vi "TwoBallAuto2safeTerminal.vi"() -> ()   [LabVIEW 2020]
uses:
  Global Variables/AutoOneBall.ctl
  Global Variables/ActuatorsSensors.vi
  <vilib>/Rock Robotics/WPI/ThirdParty/REV Robotics/REVLib/Typedef/Spark MAX Control Type.ctl
  Global Variables/Axes_N_Buttons.vi
panel:
  in  "Tab Control":T1(tab)=enum."Return Tarmac"
  out "R Output":cluster{"Applied Output":dbl}(graph)
  out "L Output":cluster{"Applied Output":dbl}(graph)
  out "PID R":cluster{"Sensor Position":dbl, "Setpoint":dbl}(graph)
  out "PID L":cluster{"Sensor Position":dbl, "Setpoint":dbl}(graph)
  in  "Reset":bool
  in  "PID Constants L":T2={"P Gain"=0.007, "I Gain"=0.0002, "D Gain"=0.0, "F Gain"=0.0, "I Zone"=1000.0, "Min Output"=-1.0, "Max Output"=1.0}
  in  "PID Constants R":T2={"P Gain"=0.003, "I Gain"=0.0002, "D Gain"=0.0, "F Gain"=0.0, "I Zone"=1000.0, "Min Output"=-0.1, "Max Output"=0.1}
  in  "Range":cluster{"output high":dbl, "output low":dbl}={"output high"=0.6, "output low"=-0.6} {"output low" format="%.2f"; "output high" format="%.2f"}
  in  "Gains":T3={"proportional gain (Kc)"=0.04, "integral time (Ti, min)"=0.0, "derivative time (Td, min)"=0.0} {"derivative time (Td, min)" format="%.3f"; "integral time (Ti, min)" format="%.3f"; "proportional gain (Kc)" format="%.3f"}
  in  "Soft start":dbl=1.8 format="%#_13g"
  in  "Meters":dbl=-2.5
  in  "Meters 2":dbl=2.3
  in  "Meters 3":dbl=-0.6
  in  "Meters 4":dbl=-0.6
  in  "Meters 5":dbl=-1.5
  in  "Meters 6":dbl=-1.0
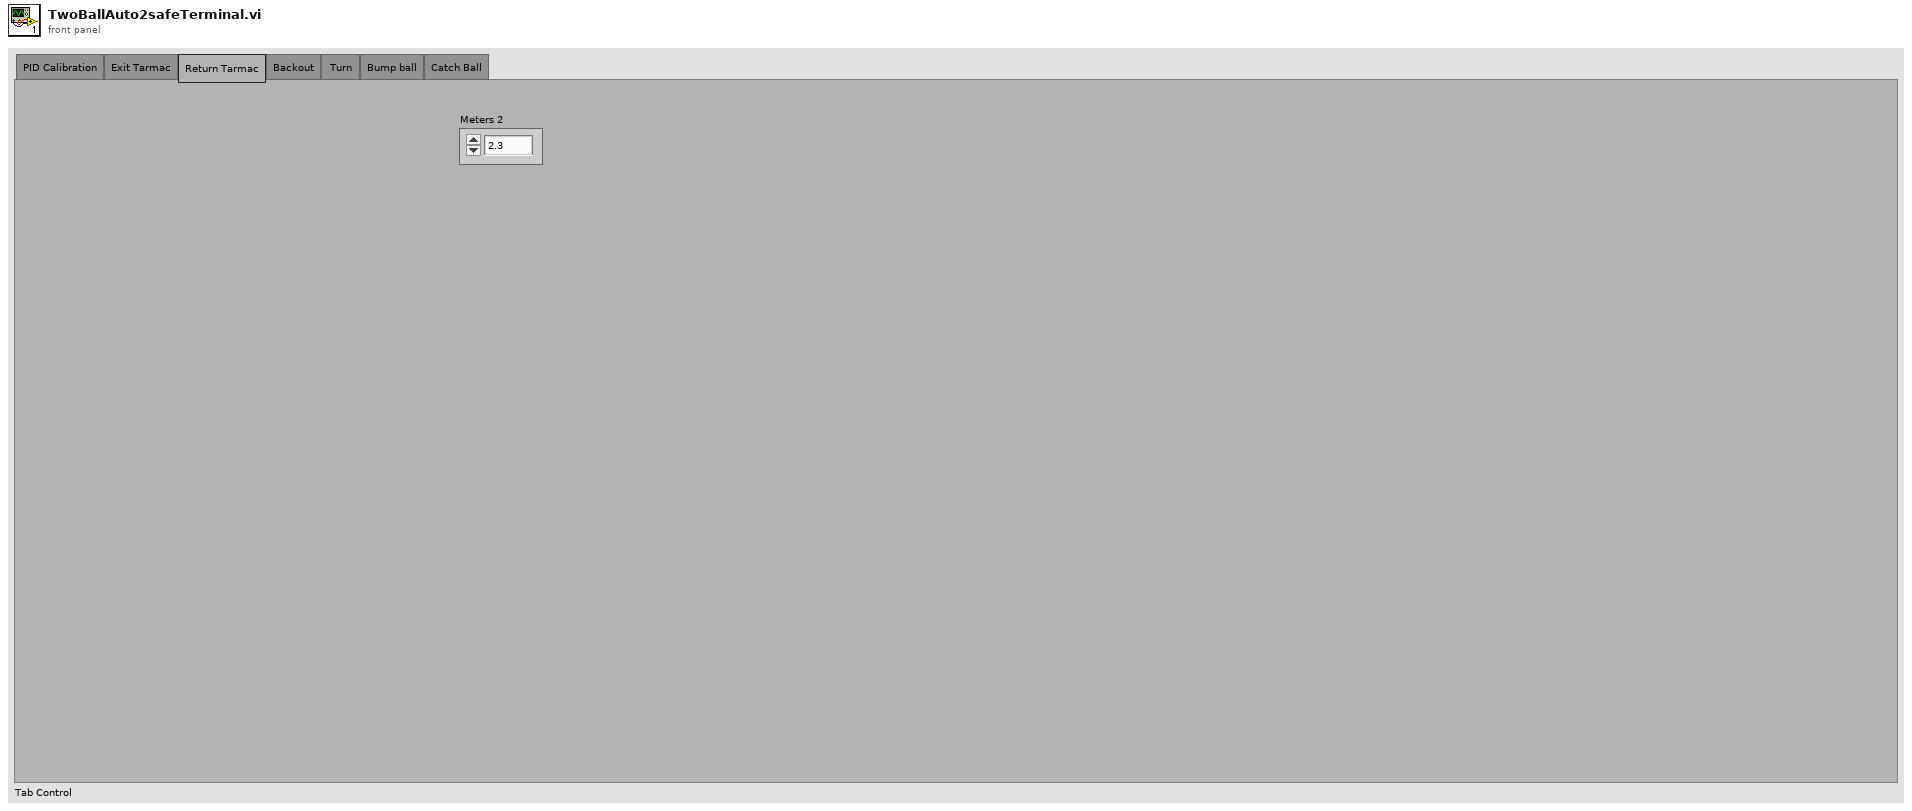
[diagram p1: front panel]
types:
  T1 = enum32{"PID Calibration", "Exit Tarmac", "Return Tarmac", "Backout", "Turn ", "Bump ball", "Catch Ball"}
  T2 = cluster{"P Gain":dbl, "I Gain":dbl, "D Gain":dbl, "F Gain":dbl, "I Zone":dbl, "Min Output":dbl, "Max Output":dbl}
  T3 = cluster{"proportional gain (Kc)":dbl, "integral time (Ti, min)":dbl, "derivative time (Td, min)":dbl}
  T4 = typedef "AutoOneBall.ctl" = enum16{"Start", "Shoot", "Delay", "Exit Tarmac", "Delay 2", "Return Tarmac", "Delay 3", "Prepare Shooter 2", "Align", "Shoot 2", "Backout", "Delay 4", "Turn", "Delay 5", "Bump Ball", "Collect Ball", "Reset"}
  T5 = typedef "WPI_MotorControlDeviceRef.ctl" = cluster{"DeviceStatus":errorcluster, "Type":T6, "PWM":cluster{"PWM Channel":T7, "DeadBand":T8}, "CAN":cluster{"Device Number":u8, "SetOutput VI Ref":variant, "GetOutput VI Ref":variant, "Enable VI Ref":variant, "Disable VI Ref":variant, "Data":variant}, "Invert":bool, "DIO PWM":cluster{"PWM \"Enable\" Channel":T7, "DIOChannel":T9, "PWM Rate":dbl}}
  T6 = typedef "WPI_MotorControlType.ctl" = enum16{"PWM", "CAN", "DIO PWM"}
  T7 = typedef "FPGA_DIOPWMChannel.ctl" = enum8{"PWM 0", "PWM 1", "PWM 2", "PWM 3", "PWM 4", "PWM 5", "PWM 6", "PWM 7", "PWM 8", "PWM 9", "PWM MXP 0", "PWM MXP 1", "PWM MXP 2", "PWM MXP 3", "PWM MXP 4", "PWM MXP 5", "PWM MXP 6", "PWM MXP 7", "PWM MXP 8", "PWM MXP 9", "Invalid"}
  T8 = typedef "WPI_PWMDeadband.ctl" = cluster{"Name":string, "maxPositivePwm":i32, "minPositivePwm":i32, "centerPwm":i32, "maxNegativePwm":i32, "minNegativePwm":i32, "angularRange":u16}
  T9 = typedef "FPGA_DIOChannel.ctl" = enum8{"DIO 0", "DIO 1", "DIO 2", "DIO 3", "DIO 4", "DIO 5", "DIO 6", "DIO 7", "DIO 8", "DIO 9", "DIO MXP 0", "DIO MXP 1", "DIO MXP 2", "DIO MXP 3", "DIO MXP 4", "DIO MXP 5", "DIO MXP 6", "DIO MXP 7", "DIO MXP 8", "DIO MXP 9", "DIO MXP 10", "DIO MXP 11", "DIO MXP 12", "DIO MXP 13", "DIO MXP 14", "DIO MXP 15", "SPI Port CS1", "SPI Port CS2", "SPI Port CS3", "SPI Port MISO", "SPI Port MOSI", "Invalid"}
  T10 = typedef "Spark MAX Control Type.ctl" = enum16{"Percent VBus", "Voltage", "Velocity", "Position", "Smart Motion", "Current", "Smart Velocity"}
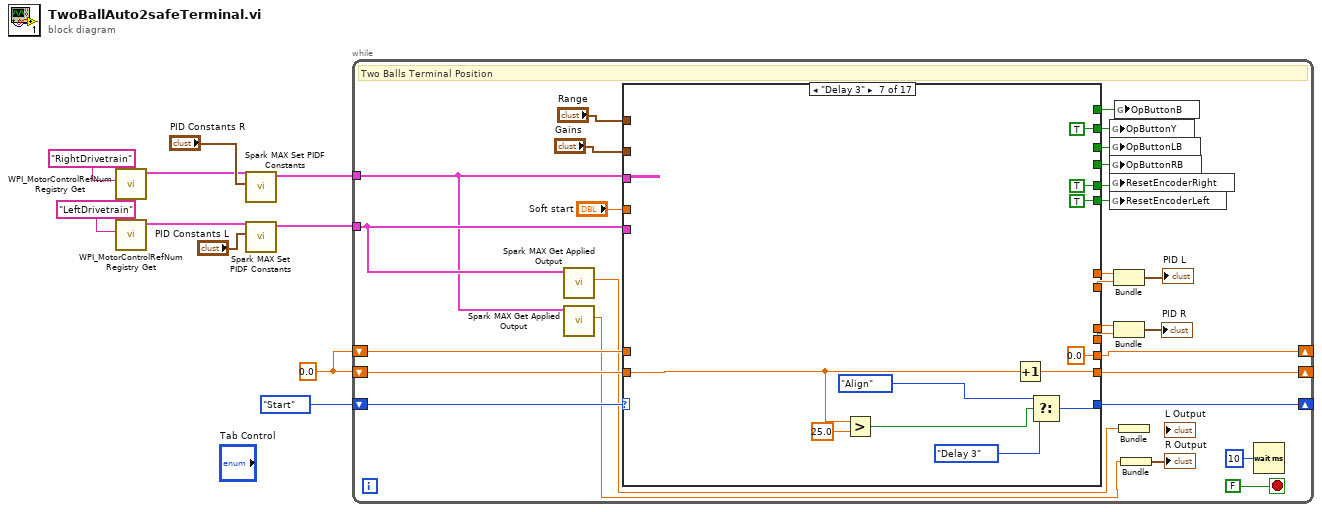
[diagram p0: block diagram]
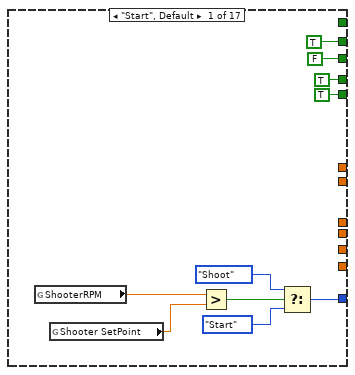
[diagram p2: hidden frame]
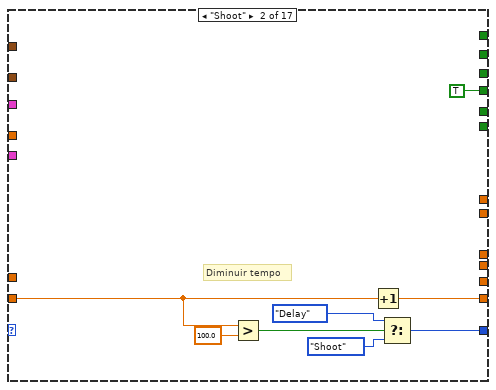
[diagram p3: hidden frame]
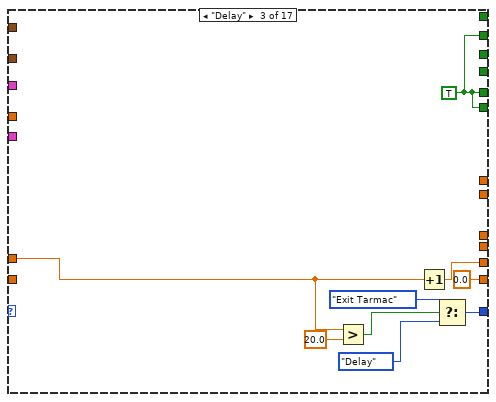
[diagram p4: hidden frame]
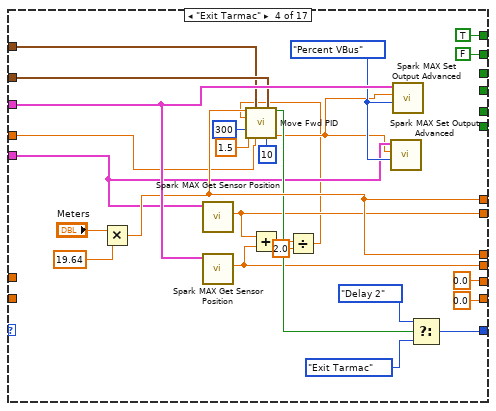
[diagram p5: hidden frame]
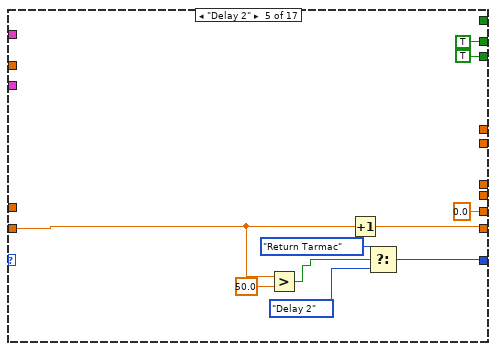
[diagram p6: hidden frame]
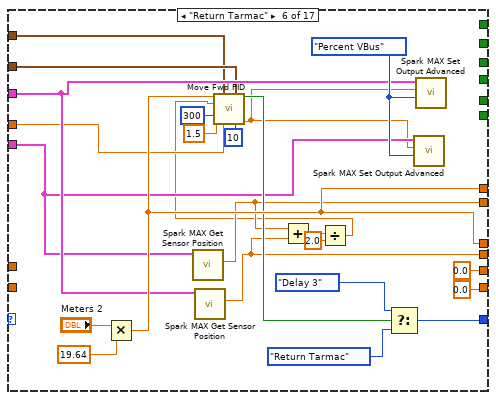
[diagram p7: hidden frame]
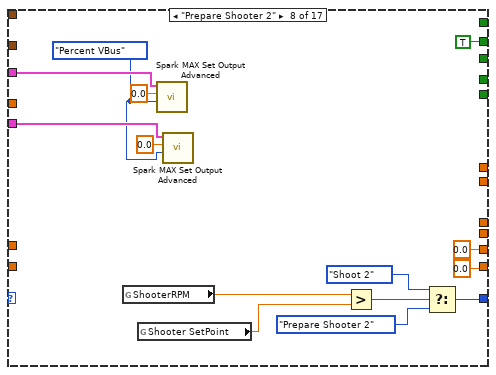
[diagram p8: hidden frame]
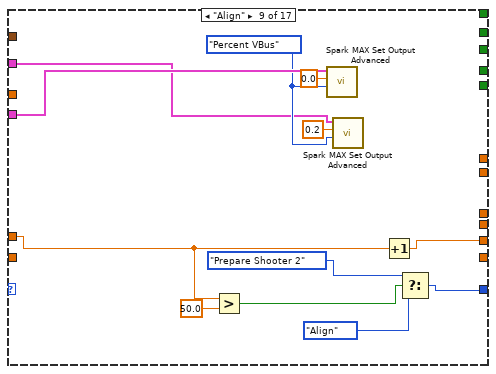
[diagram p9: hidden frame]
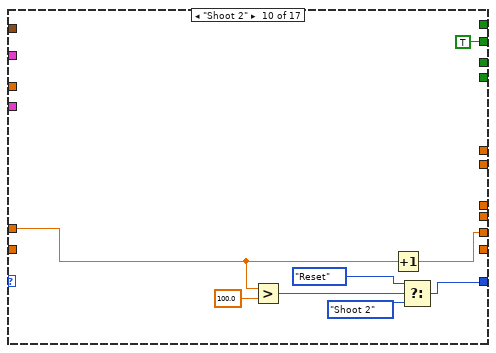
[diagram p10: hidden frame]
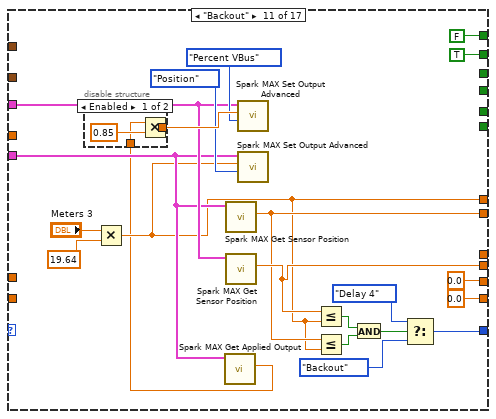
[diagram p11: hidden frame]
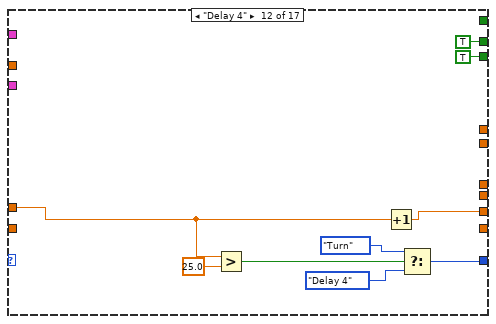
[diagram p13: hidden frame]
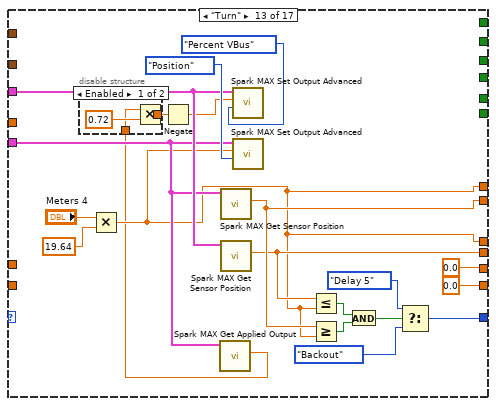
[diagram p14: hidden frame]
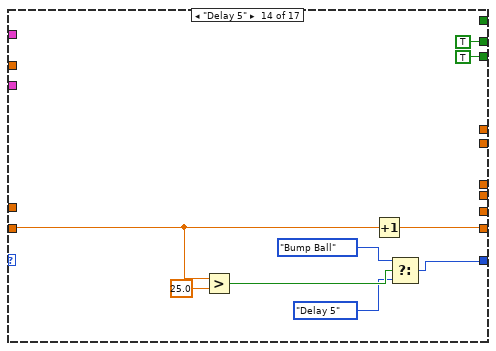
[diagram p16: hidden frame]
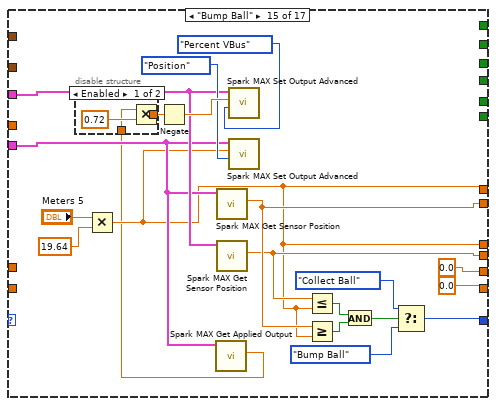
[diagram p17: hidden frame]
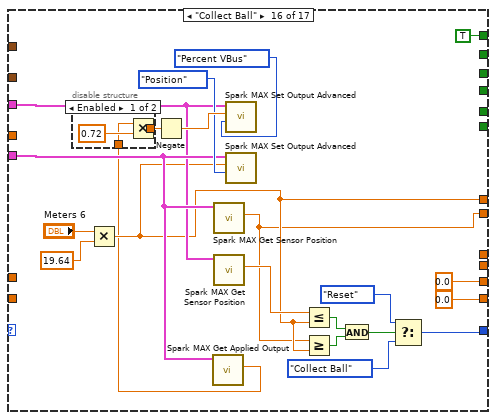
[diagram p19: hidden frame]
diagram:
  w9 = 0.0 ("Setpoint")
  n1 = call <vilib>:"WPI_MotorControlRefNum Registry Get.vi"("refnum name"="RightDrivetrain") -> ("MotorControlDevRef"=w4:T5)  [unwired: 9 in, 1 out]
  n2 = call <vilib>:"WPI_MotorControlRefNum Registry Get.vi"("refnum name"="LeftDrivetrain") -> ("MotorControlDevRef"=w3:T5)  [unwired: 9 in, 1 out]
  n3 = call <vilib>:"Spark MAX Set PIDF Constants.vi"("PID Constants"="PID Constants R", "MotorControlDeviceRef"=w4) -> ("MotorControlDeviceRef"=w1:T5)  [unwired: 8 in, 1 out]
  n4 = call <vilib>:"Spark MAX Set PIDF Constants.vi"("PID Constants"="PID Constants L", "MotorControlDeviceRef"=w3) -> ("MotorControlDeviceRef"=w2:T5)  [unwired: 8 in, 1 out]
  n5 = while {
    shift-right: [w34] -> _
    shift-left: AutoOneBall."Start" ("Enum") -> [w38]
    shift-right: [w29] -> _
    shift-left: w9 -> [w30]
    shift-right: [w20] -> _
    shift-left: w9 -> [w21]
    tunnel: w1 -> [w17]
    tunnel: w2 -> [w19]
    stop <- FALSE stop-if-true
    # "Two Balls Terminal Position"
    n6 = call <vilib>:"Spark MAX Get Applied Output.vi"("MotorControlDevRef in"=w19) -> ("Applied Output"=w13:dbl)  [unwired: 7 in, 3 out]
    n7 = call <vilib>:"Spark MAX Get Applied Output.vi"("MotorControlDevRef in"=w17) -> ("Applied Output"=w16:dbl)  [unwired: 7 in, 3 out]
    n8 = case shown="\"Delay 3\"" w38 {
      tunnel: w19 -> [_ _ _ w77 _ w112 _ w138 w162 _ w180 _ w214 _ w245 w269 _]
      tunnel: w17 -> [_ _ _ w83 _ w113 _ w139 w153 _ w181 _ w215 _ w246 w268 _]
      tunnel: [TRUE ("OpButtonLB") _ _ _ _ _ _ TRUE ("OpButtonLB") _ _ _ _ _ _ _ _ _] -> w35
      tunnel: [w43 w49 w64 w89 w96 w124 w129 w145 w156 w166 w174 w198 w208 w231 w241 w270 w291] -> w34
      tunnel: [_ _ _ w70 _ w104 _ _ _ _ w176 _ w213 _ w244 w266 _] -> w22
      tunnel: [_ _ _ w69 _ w105 _ _ _ _ w177 _ w210 _ w243 _ _] -> w24
      tunnel: [_ _ _ w79 _ w115 _ _ _ _ w175 _ w209 _ w242 w267 _] -> w23
      tunnel: [_ _ _ w79 _ w115 _ _ _ _ _ _ w209 _ w242 _ _] -> w25
      tunnel: [FALSE ("DrButtonRB") TRUE ("DrButtonRB") _ _ _ _ _ _ _ TRUE ("DrButtonRB") _ _ _ _ _ _ _] -> w31
      tunnel: w30 -> [_ w55 _ _ w98 _ w135 _ _ _ _ _ _ w233 _ _ _]
      tunnel: [_ w53 0.0 0.0 w97 0.0 w133 0.0 _ _ 0.0 _ 0.0 w232 0.0 0.0 _] -> w29
      tunnel: [TRUE ("ResetEncoderRight") _ w60 _ TRUE ("ResetEncoderRight") _ TRUE ("ResetEncoderRight") _ _ _ _ TRUE ("ResetEncoderRight") _ TRUE ("ResetEncoderRight") _ _ TRUE ("ResetEncoderRight")] -> w28
      tunnel: [TRUE ("ResetEncoderRight") _ w60 _ TRUE ("ResetEncoderRight") _ TRUE ("ResetEncoderRight") _ _ _ _ TRUE ("ResetEncoderRight") _ TRUE ("ResetEncoderRight") _ _ TRUE ("ResetEncoderRight")] -> w27
      tunnel: [_ _ w60 FALSE ("ResetEncoderRight") _ _ TRUE ("ResetEncoderRight") _ _ _ TRUE ("ResetEncoderRight") _ _ _ _ _ TRUE ("ResetEncoderRight")] -> w26
      tunnel: w21 -> [_ _ w59 _ _ _ _ _ w152 w164 _ w200 _ _ _ _ _]
      tunnel: [_ _ w58 0.0 0.0 0.0 0.0 0.0 w151 w163 0.0 w199 0.0 _ 0.0 0.0 _] -> w20
      tunnel: [_ _ _ TRUE ("ResetEncoderRight") _ _ _ _ _ _ FALSE ("ResetEncoderRight") _ _ _ _ TRUE ("ResetEncoderRight") _] -> w18
      tunnel: "Soft start" -> [_ _ _ w74 _ w111 _ _ _ _ _ _ _ _ _ _ _]
      tunnel: "Gains" -> [_ _ _ w73 _ w110 _ _ _ _ _ _ _ _ _ _ _]
      tunnel: "Range" -> [_ _ _ w72 _ w109 _ _ _ _ _ _ _ _ _ _ _]
      frame "Start", Default {
        n9 = global read "ActuatorsSensors.vi" "ShooterRPM"() -> (w47:dbl)
        n10 = global read "ActuatorsSensors.vi" "Shooter SetPoint"() -> (w39:dbl)
        n11 = Greater?(x=w47, y=w39) -> (0:w46:bool)
        n12 = Select(t=AutoOneBall."Shoot" ("Enum"), s=w46, f=AutoOneBall."Start" ("Enum")) -> (s? t:f=w43:T4)
      }
      frame "Shoot" {
        # "Diminuir tempo"
        n13 = Greater?(x=w55, y=100.0) -> (0:w52:bool)
        n14 = Increment(x=w55) -> (x+1=w53:dbl)
        n15 = Select(t=AutoOneBall."Delay" ("Enum"), s=w52, f=AutoOneBall."Shoot" ("Enum")) -> (s? t:f=w49:T4)
      }
      frame "Delay" {
        w60 = TRUE ("ResetEncoderRight")
        n16 = Greater?(x=w59, y=20.0) -> (0:w63:bool)
        n17 = Increment(x=w59) -> (x+1=w58:dbl)
        n18 = Select(t=AutoOneBall."Exit Tarmac" ("Enum"), s=w63, f=AutoOneBall."Delay" ("Enum")) -> (s? t:f=w64:T4)
      }
      frame "Exit Tarmac" {
        w80 = Spark_MAX_Control_Type."Percent VBus" ("Control Mode")
        n19 = Multiply(x="Meters", y=19.64) -> (x*y=w79:dbl)
        n20 = call <vilib>:"Spark MAX Get Sensor Position.vi"("MotorControlDevRef in"=w77) -> ("Sensor Position"=w70:dbl)  [unwired: 7 in, 3 out]
        n21 = call <vilib>:"Spark MAX Get Sensor Position.vi"("MotorControlDevRef in"=w83) -> ("Sensor Position"=w69:dbl)  [unwired: 7 in, 3 out]
        n22 = Add(x=w70, y=w69) -> (x+y=w68:dbl)
        n23 = Divide(x=w68, y=2.0) -> (x/y=w66:dbl)
        n24 = call "Move Fwd PID.vi"("Distance"=w79, "Range"=w72, "Gains"=w73, "Encoder Count"=w66, "Time to stop"=300, "Precision"=1.5, "Soft start"=w74, "Loop Timer"=10) -> ("Finished?"=w78:bool, "Output"=w75:dbl)  [unwired: 6 in]
        n25 = call <vilib>:"Spark MAX Set Output Advanced.vi"("Control Mode"=w80, "Setpoint"=w75, "MotorControlDevRef"=w77) -> ()  [unwired: 7 in, 2 out]
        n26 = call <vilib>:"Spark MAX Set Output Advanced.vi"("Control Mode"=w80, "Setpoint"=w75, "MotorControlDevRef"=w83) -> ()  [unwired: 7 in, 2 out]
        n27 = Select(t=AutoOneBall."Delay 2" ("Enum"), s=w78, f=AutoOneBall."Exit Tarmac" ("Enum")) -> (s? t:f=w89:T4)
      }
      frame "Delay 2" {
        n28 = Greater?(x=w98, y=50.0) -> (0:w94:bool)
        n29 = Increment(x=w98) -> (x+1=w97:dbl)
        n30 = Select(t=AutoOneBall."Return Tarmac" ("Enum"), s=w94, f=AutoOneBall."Delay 2" ("Enum")) -> (s? t:f=w96:T4)
      }
      frame "Return Tarmac" {
        w116 = Spark_MAX_Control_Type."Percent VBus" ("Control Mode")
        n31 = Multiply(x="Meters 2", y=19.64) -> (x*y=w115:dbl)
        n32 = call <vilib>:"Spark MAX Get Sensor Position.vi"("MotorControlDevRef in"=w112) -> ("Sensor Position"=w104:dbl)  [unwired: 7 in, 3 out]
        n33 = call <vilib>:"Spark MAX Get Sensor Position.vi"("MotorControlDevRef in"=w113) -> ("Sensor Position"=w105:dbl)  [unwired: 7 in, 3 out]
        n34 = Add(x=w104, y=w105) -> (x+y=w103:dbl)
        n35 = Divide(x=w103, y=2.0) -> (x/y=w102:dbl)
        n36 = call "Move Fwd PID.vi"("Distance"=w115, "Range"=w109, "Gains"=w110, "Encoder Count"=w102, "Time to stop"=300, "Precision"=1.5, "Soft start"=w111, "Loop Timer"=10) -> ("Finished?"=w114:bool, "Output"=w107:dbl)  [unwired: 6 in]
        n37 = Select(t=AutoOneBall."Delay 3" ("Enum"), s=w114, f=AutoOneBall."Return Tarmac" ("Enum")) -> (s? t:f=w124:T4)
        n38 = call <vilib>:"Spark MAX Set Output Advanced.vi"("Control Mode"=w116, "Setpoint"=w107, "MotorControlDevRef"=w112) -> ()  [unwired: 7 in, 2 out]
        n39 = call <vilib>:"Spark MAX Set Output Advanced.vi"("Control Mode"=w116, "Setpoint"=w107, "MotorControlDevRef"=w113) -> ()  [unwired: 7 in, 2 out]
      }
      frame "Delay 3" {
        n40 = Greater?(x=w135, y=25.0) -> (0:w132:bool)
        n41 = Increment(x=w135) -> (x+1=w133:dbl)
        n42 = Select(t=AutoOneBall."Align" ("Enum"), s=w132, f=AutoOneBall."Delay 3" ("Enum")) -> (s? t:f=w129:T4)
      }
      frame "Prepare Shooter 2" {
        w137 = Spark_MAX_Control_Type."Percent VBus" ("Control Mode")
        n43 = global read "ActuatorsSensors.vi" "ShooterRPM"() -> (w148:dbl)
        n44 = global read "ActuatorsSensors.vi" "Shooter SetPoint"() -> (w150:dbl)
        n45 = call <vilib>:"Spark MAX Set Output Advanced.vi"("Control Mode"=w137, "Setpoint"=0.0, "MotorControlDevRef"=w139) -> ()  [unwired: 7 in, 2 out]
        n46 = call <vilib>:"Spark MAX Set Output Advanced.vi"("Control Mode"=w137, "Setpoint"=0.0, "MotorControlDevRef"=w138) -> ()  [unwired: 7 in, 2 out]
        n47 = Greater?(x=w148, y=w150) -> (0:w149:bool)
        n48 = Select(t=AutoOneBall."Shoot 2" ("Enum"), s=w149, f=AutoOneBall."Prepare Shooter 2" ("Enum")) -> (s? t:f=w145:T4)
      }
      frame "Align" {
        w154 = Spark_MAX_Control_Type."Percent VBus" ("Control Mode")
        n49 = Greater?(x=w152, y=50.0) -> (0:w159:bool)
        n50 = call <vilib>:"Spark MAX Set Output Advanced.vi"("Control Mode"=w154, "Setpoint"=0.0, "MotorControlDevRef"=w162) -> ()  [unwired: 7 in, 2 out]
        n51 = call <vilib>:"Spark MAX Set Output Advanced.vi"("Control Mode"=w154, "Setpoint"=0.2, "MotorControlDevRef"=w153) -> ()  [unwired: 7 in, 2 out]
        n52 = Increment(x=w152) -> (x+1=w151:dbl)
        n53 = Select(t=AutoOneBall."Prepare Shooter 2" ("Enum"), s=w159, f=AutoOneBall."Align" ("Enum")) -> (s? t:f=w156:T4)
      }
      frame "Shoot 2" {
        n54 = Greater?(x=w164, y=100.0) -> (0:w169:bool)
        n55 = Increment(x=w164) -> (x+1=w163:dbl)
        n56 = Select(t=AutoOneBall."Reset" ("Enum"), s=w169, f=AutoOneBall."Shoot 2" ("Enum")) -> (s? t:f=w166:T4)
      }
      frame "Backout" {
        n57 = Multiply(x="Meters 3", y=19.64) -> (x*y=w175:dbl)
        n58 = call <vilib>:"Spark MAX Get Applied Output.vi"("MotorControlDevRef in"=w180) -> ("Applied Output"=w171:dbl)  [unwired: 7 in, 3 out]
        n59 = disable-structure shown="Enabled" {
          disable-tunnel: w171 -> [w193 w195]
          disable-tunnel: [w192 w195] -> w190
          frame Enabled {
            n60 = Multiply(x=w193, y=0.85) -> (x*y=w192:dbl)
          }
          frame Disabled {
          }
        }
        n61 = call <vilib>:"Spark MAX Get Sensor Position.vi"("MotorControlDevRef in"=w180) -> ("Sensor Position"=w176:dbl)  [unwired: 7 in, 3 out]
        n62 = call <vilib>:"Spark MAX Get Sensor Position.vi"("MotorControlDevRef in"=w181) -> ("Sensor Position"=w177:dbl)  [unwired: 7 in, 3 out]
        n63 = call <vilib>:"Spark MAX Set Output Advanced.vi"("Control Mode"=Spark_MAX_Control_Type."Percent VBus", "Setpoint"=w190, "MotorControlDevRef"=w181) -> ()  [unwired: 7 in, 2 out]
        n64 = call <vilib>:"Spark MAX Set Output Advanced.vi"("Control Mode"=Spark_MAX_Control_Type."Position", "Setpoint"=w175, "MotorControlDevRef"=w180) -> ()  [unwired: 7 in, 2 out]
        n65 = Less Or Equal?(x=w177, y=w175) -> (x <= y?=w187:bool)
        n66 = Less Or Equal?(x=w176, y=w175) -> (x <= y?=w188:bool)
        n67 = And(x=w187, y=w188) -> (x .and. y?=w189:bool)
        n68 = Select(t=AutoOneBall."Delay 4" ("Enum"), s=w189, f=AutoOneBall."Backout" ("Enum")) -> (s? t:f=w174:T4)
      }
      frame "Delay 4" {
        n69 = Greater?(x=w200, y=25.0) -> (0:w204:bool)
        n70 = Increment(x=w200) -> (x+1=w199:dbl)
        n71 = Select(t=AutoOneBall."Turn" ("Enum"), s=w204, f=AutoOneBall."Delay 4" ("Enum")) -> (s? t:f=w198:T4)
      }
      frame "Turn" {
        n72 = Multiply(x="Meters 4", y=19.64) -> (x*y=w209:dbl)
        n73 = call <vilib>:"Spark MAX Get Applied Output.vi"("MotorControlDevRef in"=w214) -> ("Applied Output"=w205:dbl)  [unwired: 7 in, 3 out]
        n74 = disable-structure shown="Enabled" {
          disable-tunnel: w205 -> [w226 w228]
          disable-tunnel: [w225 w228] -> w207
          frame Enabled {
            n75 = Multiply(x=w226, y=0.72) -> (x*y=w225:dbl)
          }
          frame Disabled {
          }
        }
        n76 = Negate(x=w207) -> (-x=w206:dbl)
        n77 = call <vilib>:"Spark MAX Get Sensor Position.vi"("MotorControlDevRef in"=w214) -> ("Sensor Position"=w213:dbl)  [unwired: 7 in, 3 out]
        n78 = call <vilib>:"Spark MAX Get Sensor Position.vi"("MotorControlDevRef in"=w215) -> ("Sensor Position"=w210:dbl)  [unwired: 7 in, 3 out]
        n79 = call <vilib>:"Spark MAX Set Output Advanced.vi"("Control Mode"=Spark_MAX_Control_Type."Percent VBus", "Setpoint"=w206, "MotorControlDevRef"=w215) -> ()  [unwired: 7 in, 2 out]
        n80 = call <vilib>:"Spark MAX Set Output Advanced.vi"("Control Mode"=Spark_MAX_Control_Type."Position", "Setpoint"=w209, "MotorControlDevRef"=w214) -> ()  [unwired: 7 in, 2 out]
        n81 = Less Or Equal?(x=w210, y=w209) -> (x <= y?=w224:bool)
        n82 = Greater Or Equal?(x=w213, y=w209) -> (x >= y?=w223:bool)
        n83 = And(x=w224, y=w223) -> (x .and. y?=w222:bool)
        n84 = Select(t=AutoOneBall."Delay 5" ("Enum"), s=w222, f=AutoOneBall."Backout" ("Enum")) -> (s? t:f=w208:T4)
      }
      frame "Delay 5" {
        n85 = Greater?(x=w233, y=25.0) -> (0:w237:bool)
        n86 = Increment(x=w233) -> (x+1=w232:dbl)
        n87 = Select(t=AutoOneBall."Bump Ball" ("Enum"), s=w237, f=AutoOneBall."Delay 5" ("Enum")) -> (s? t:f=w231:T4)
      }
      frame "Bump Ball" {
        n88 = Multiply(x="Meters 5", y=19.64) -> (x*y=w242:dbl)
        n89 = call <vilib>:"Spark MAX Get Applied Output.vi"("MotorControlDevRef in"=w245) -> ("Applied Output"=w238:dbl)  [unwired: 7 in, 3 out]
        n90 = disable-structure shown="Enabled" {
          disable-tunnel: w238 -> [w259 w261]
          disable-tunnel: [w258 w261] -> w256
          frame Enabled {
            n91 = Multiply(x=w259, y=0.72) -> (x*y=w258:dbl)
          }
          frame Disabled {
          }
        }
        n92 = Negate(x=w256) -> (-x=w257:dbl)
        n93 = call <vilib>:"Spark MAX Get Sensor Position.vi"("MotorControlDevRef in"=w245) -> ("Sensor Position"=w244:dbl)  [unwired: 7 in, 3 out]
        n94 = call <vilib>:"Spark MAX Get Sensor Position.vi"("MotorControlDevRef in"=w246) -> ("Sensor Position"=w243:dbl)  [unwired: 7 in, 3 out]
        n95 = call <vilib>:"Spark MAX Set Output Advanced.vi"("Control Mode"=Spark_MAX_Control_Type."Percent VBus", "Setpoint"=w257, "MotorControlDevRef"=w246) -> ()  [unwired: 7 in, 2 out]
        n96 = call <vilib>:"Spark MAX Set Output Advanced.vi"("Control Mode"=Spark_MAX_Control_Type."Position", "Setpoint"=w242, "MotorControlDevRef"=w245) -> ()  [unwired: 7 in, 2 out]
        n97 = Less Or Equal?(x=w243, y=w242) -> (x <= y?=w252:bool)
        n98 = Greater Or Equal?(x=w244, y=w242) -> (x >= y?=w253:bool)
        n99 = And(x=w252, y=w253) -> (x .and. y?=w254:bool)
        n100 = Select(t=AutoOneBall."Collect Ball" ("Enum"), s=w254, f=AutoOneBall."Bump Ball" ("Enum")) -> (s? t:f=w241:T4)
      }
      frame "Collect Ball" {
        n101 = Multiply(x="Meters 6", y=19.64) -> (x*y=w267:dbl)
        n102 = call <vilib>:"Spark MAX Get Applied Output.vi"("MotorControlDevRef in"=w269) -> ("Applied Output"=w262:dbl)  [unwired: 7 in, 3 out]
        n103 = disable-structure shown="Enabled" {
          disable-tunnel: w262 -> [w284 w286]
          disable-tunnel: [w283 w286] -> w281
          frame Enabled {
            n104 = Multiply(x=w284, y=0.72) -> (x*y=w283:dbl)
          }
          frame Disabled {
          }
        }
        n105 = Negate(x=w281) -> (-x=w282:dbl)
        n106 = call <vilib>:"Spark MAX Get Sensor Position.vi"("MotorControlDevRef in"=w269) -> ("Sensor Position"=w266:dbl)  [unwired: 7 in, 3 out]
        n107 = call <vilib>:"Spark MAX Get Sensor Position.vi"("MotorControlDevRef in"=w268) -> ("Sensor Position"=w280:dbl)  [unwired: 7 in, 3 out]
        n108 = call <vilib>:"Spark MAX Set Output Advanced.vi"("Control Mode"=Spark_MAX_Control_Type."Percent VBus", "Setpoint"=w282, "MotorControlDevRef"=w268) -> ()  [unwired: 7 in, 2 out]
        n109 = call <vilib>:"Spark MAX Set Output Advanced.vi"("Control Mode"=Spark_MAX_Control_Type."Position", "Setpoint"=w267, "MotorControlDevRef"=w269) -> ()  [unwired: 7 in, 2 out]
        n110 = Less Or Equal?(x=w280, y=w267) -> (x <= y?=w276:bool)
        n111 = Greater Or Equal?(x=w266, y=w267) -> (x >= y?=w277:bool)
        n112 = And(x=w276, y=w277) -> (x .and. y?=w278:bool)
        n113 = Select(t=AutoOneBall."Reset" ("Enum"), s=w278, f=AutoOneBall."Collect Ball" ("Enum")) -> (s? t:f=w270:T4)
      }
      frame "Reset" {
        n114 = Select(t=AutoOneBall."Start" ("Enum"), s="Reset", f=AutoOneBall."Reset" ("Enum")) -> (s? t:f=w291:T4)
      }
    }
    n115 = global write "Axes_N_Buttons.vi" "OpButtonY"(w26) -> ()
    n116 = global write "Axes_N_Buttons.vi" "OpButtonLB"(w35) -> ()
    n117 = global write "Axes_N_Buttons.vi" "OpButtonRB"(w31) -> ()
    n118 = global write "ActuatorsSensors.vi" "ResetEncoderRight"(w28) -> ()
    n119 = global write "ActuatorsSensors.vi" "ResetEncoderLeft"(w27) -> ()
    n120 = Bundle(w23, "Sensor Position"=w22) -> (→"PID L":cluster{dbl, "Sensor Position":dbl})  [unwired: 1 in]
    n121 = Bundle(w25, "Sensor Position"=w24) -> (→"PID R":cluster{dbl, "Sensor Position":dbl})  [unwired: 1 in]
    n122 = global write "Axes_N_Buttons.vi" "OpButtonB"(w18) -> ()
    n123 = Bundle("Applied Output"=w13) -> ()  [unwired: 1 in, 1 out]
    n124 = Bundle("Applied Output"=w16) -> (→"R Output":cluster{"Applied Output":dbl})  [unwired: 1 in]
    n125 = Wait (ms)(milliseconds to wait=u32 10) -> ()  [unwired: 1 out]
  }
